vi "Read_Instr.vi"(8 "error in (no error)":errorcluster caption="entrée d'erreur (pas d'erreur)", 11 "Class Instrument Firebase en entrée":refnum<class "Class Instrument Database Altyor.lvclass">) -> (0 "error out":errorcluster caption="sortie d'erreur", 3 "Class Instrument Firebase en sortie":refnum<class "Class Instrument Database Altyor.lvclass">)   [LabVIEW 2020, in "Library Instrument & Equipement.lvlib" / "Library Instruments.lvlib" / "Class Instrument Database Altyor.lvclass"]
uses:
  Class Instrument Database Altyor.lvclass
  Class Instrument Database Altyor.lvclass/Class Instrument Database Altyor.ctl
  Instrument (Default)/Class Instrument (Default).lvclass
  Database/Database Altyor/Database Altyor.lvclass
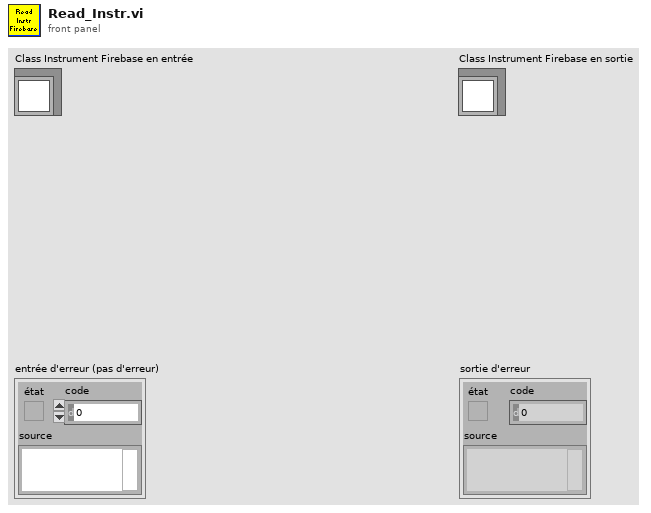
[diagram p1: front panel]
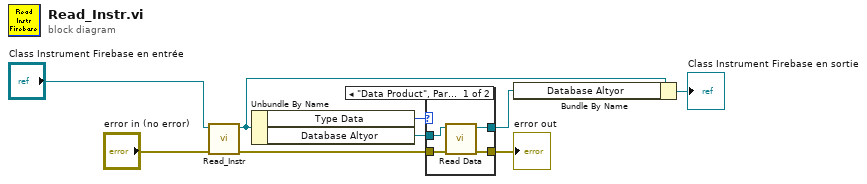
[diagram p0: block diagram]
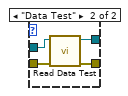
[diagram p2: hidden frame]
diagram:
  n1 = call-parent "Read_Instr.vi"("error in (no error)"="error in (no error)", "Class Instrument (Default) en entrée"="Class Instrument Firebase en entrée") -> ("error out"=w5:errorcluster, "Class Instrument (Default) en sortie"=w3:refnum<class "Class Instrument Database Altyor.lvclass">)  [unwired: 8 in]
  n2 = Unbundle By Name(w3) -> ("Type Data"=w7:enum16{"Data Product", "Data Test"}, "Database Altyor"=w6:refnum<class "Database Altyor.lvclass">)
  n3 = case shown="\"Data Product\", Par défaut" w7 {
    tunnel: w5 -> [w10 w17]
    tunnel: [w13 w16] -> w4
    tunnel: w6 -> [w11 w14]
    tunnel: [w12 w15] -> w1
    frame "Data Product", Default {
      n4 = call-dynamic "Read Data.vi"("error in (no error)"=w10, "Database Altyor en entrée"=w11) -> ("error out"=w13:errorcluster, "Database Altyor en sortie"=w12:refnum<class "Database Altyor.lvclass">)  [unwired: 8 in]
    }
    frame "Data Test" {
      n5 = call-dynamic "Read Data Test.vi"("error in (no error)"=w17, "Database Altyor en entrée"=w14) -> ("error out"=w16:errorcluster, "Database Altyor en sortie"=w15:refnum<class "Database Altyor.lvclass">)  [unwired: 8 in]
    }
  }
  "error out" <- w4
  n6 = Bundle By Name(cluster=w3, "Database Altyor"=w1) -> (→"Class Instrument Firebase en sortie":refnum<class "Class Instrument Database Altyor.lvclass">)
